vi "Test Bench v14 - TDMS.vi"() -> ()   [LabVIEW 2022 SP3]
uses:
  WhiteNoise.ctl
  <vilib>/Utility/error.llb/DialogType.ctl
  <vilib>/Platform/TimedLoop/XDataNode/timing_clust.ctl
  <vilib>/Platform/TimedLoop/XDataNode/nitl_modes.ctl
  <vilib>/Platform/TimedLoop/XDataNode/wakeup.ctl
  <vilib>/DAQmx/write.llb/DAQmx Write (Analog 2D DBL NChan NSamp).vi
  <vilib>/DAQmx/read.llb/DAQmx Read (Analog 1D DBL 1Chan NSamp).vi
  <vilib>/DAQmx/create/channels.llb/DAQmx Create Channel (AI-Acceleration-Accelerometer).vi
  <vilib>/DAQmx/create/channels.llb/DAQmx Create Channel (AO-Voltage-Basic).vi
  <vilib>/DAQmx/configure/timing.llb/DAQmx Timing (Sample Clock).vi
  <vilib>/DAQmx/miscellaneous.llb/DAQmx Fill In Error Info.vi
  <vilib>/Platform/TimedLoop/TimeConversion.llb/rt-milliseconds-to-timestamp.vi
  <vilib>/platform/TimedLoop/XDataNode/XDataNode.xnode
  <resource>/objmgr/daqmx.rc
  <vilib>/measure/NI_MABase.lvlib
  <vilib>/Platform/TimedLoop/XDataNode/XDNodeRunTimeDep.lvlib
panel:
  in  "stop":bool
  out "x/y":dbl
  out "SampClk.Rate":dbl
  out "Accel. 1 Raw":dbl[](graph)
  in  "Enable Display":bool=TRUE
  in  "Folder to save file to":path=path "C:/Users/LAV-UFSC-2023/Documents/LAV-TCC/Dados-Experimentos/Dados-Bancada-LABVIEW"
  out "Output Signal":dynamicdata(graph)
  in  "Accel. 2":bool
  in  "Input":bool=TRUE
  out "New file path":path
  in  "Signal Output\nControl":enum32{"White Noise", "Harmonic"}(tab)
  in  "White Noise\nParameters":T2={"Seed"=0.0, "Standard Deviation"=0.2, "Reset"=FALSE, "Iterator"=1.0, "Seed"=-1, "Lower Cut-Off"=5.0, "Upper Cut-Off"=350.0} {"Upper Cut-Off" min=5.0 max=350.0 step=10.0; "Lower Cut-Off" min=5.0 max=350.0 step=10.0; "Standard Deviation" min=0.001 max=3.0 step=0.05 format="%0.2p"}
  out "dt White Noise":dbl
  in  "Hamonic\nParameters":T3={"Waveform Type"=0, "Frequency"=10.0, "Amplitude"=0.25} {"Frequency" min=5.0 max=350.0 step=10.0 format="%0.2p"; "Waveform Type" items=["Sine Wave", "Triangle Wave", "Square Wave", "Sawtooth Wave"]; "Amplitude" min=0.001 max=0.3 step=0.05 format="%0.2p"}
  out "dt Harmonic":dbl
  in  "Output":bool=TRUE
  # "Filter"
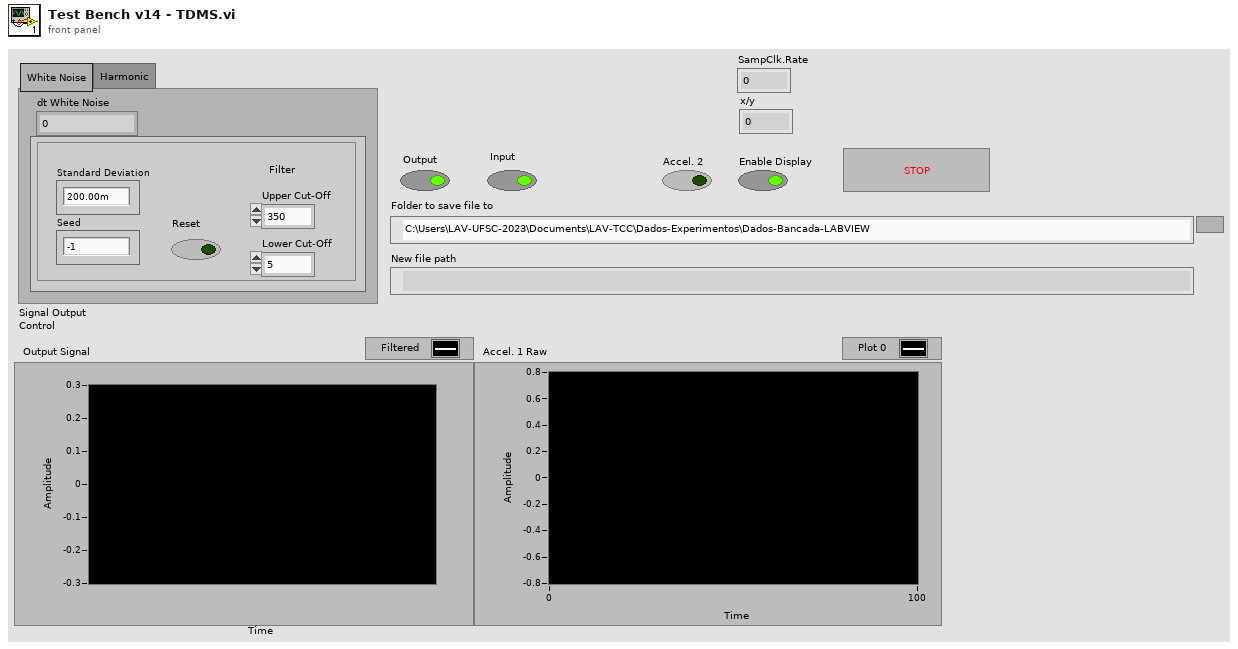
[diagram p1: front panel]
types:
  T1 = typedef "WhiteNoise.ctl" = dbl
  T2 = cluster{"Seed":T1, "Standard Deviation":dbl, "Reset":bool, "Iterator":dbl, "Seed":i8, "Lower Cut-Off":dbl, "Upper Cut-Off":dbl}
  T3 = cluster{"Waveform Type":u16, "Frequency":dbl, "Amplitude":dbl}
  T4 = enum16{"open", "open or create", "create or replace", "create", "open (read-only)"}
  T5 = typedef "DialogType.ctl" = u16
  T6 = typedef "XDNodeRunTimeDep.lvlib/timing_clust.ctl" = cluster{"Expected End [f-1]":u64, "Actual End [f-1]":u64, "Finished Late? [f-1]":bool, "Expected End [i-1]":u64, "Actual End [i-1]":u64, "Finished Late? [i-1]":bool, "Expected Start [i]":u64, "Actual Start [i]":u64, "Expected Start [f]":u64, "Actual Start [f]":u64, "Source Name":string, "Structure Name":string, "Period":i64, "Deadline":i64, "Offset":i64, "Start":i64, "Priority":i32, "Timeout":i32, "Mode":T7, "Wakeup Reason":T8, "Error":errorcluster, "Source Type":string, "Secondary Source Type":string, "Global End Time":u64, "Global Start Time":u64, "Frame Duration":u64, "Iteration Duration":u64, "Assigned CPU":i32, "I/O Scan Engine Mode":u32}
  T7 = typedef "XDNodeRunTimeDep.lvlib/nitl_modes.ctl" = enum32{"No Change", "Process missed periods, maintain original phase", "Discard missed periods, maintain original phase", "Process missed periods, ignore original phase", "Discard missed periods, ignore original phase"}
  T8 = typedef "XDNodeRunTimeDep.lvlib/wakeup.ctl" = enum32{"Normal", "Aborted", "Asynchronous wakeup", "Timing source error", "Timed loop error", "Timeout"}
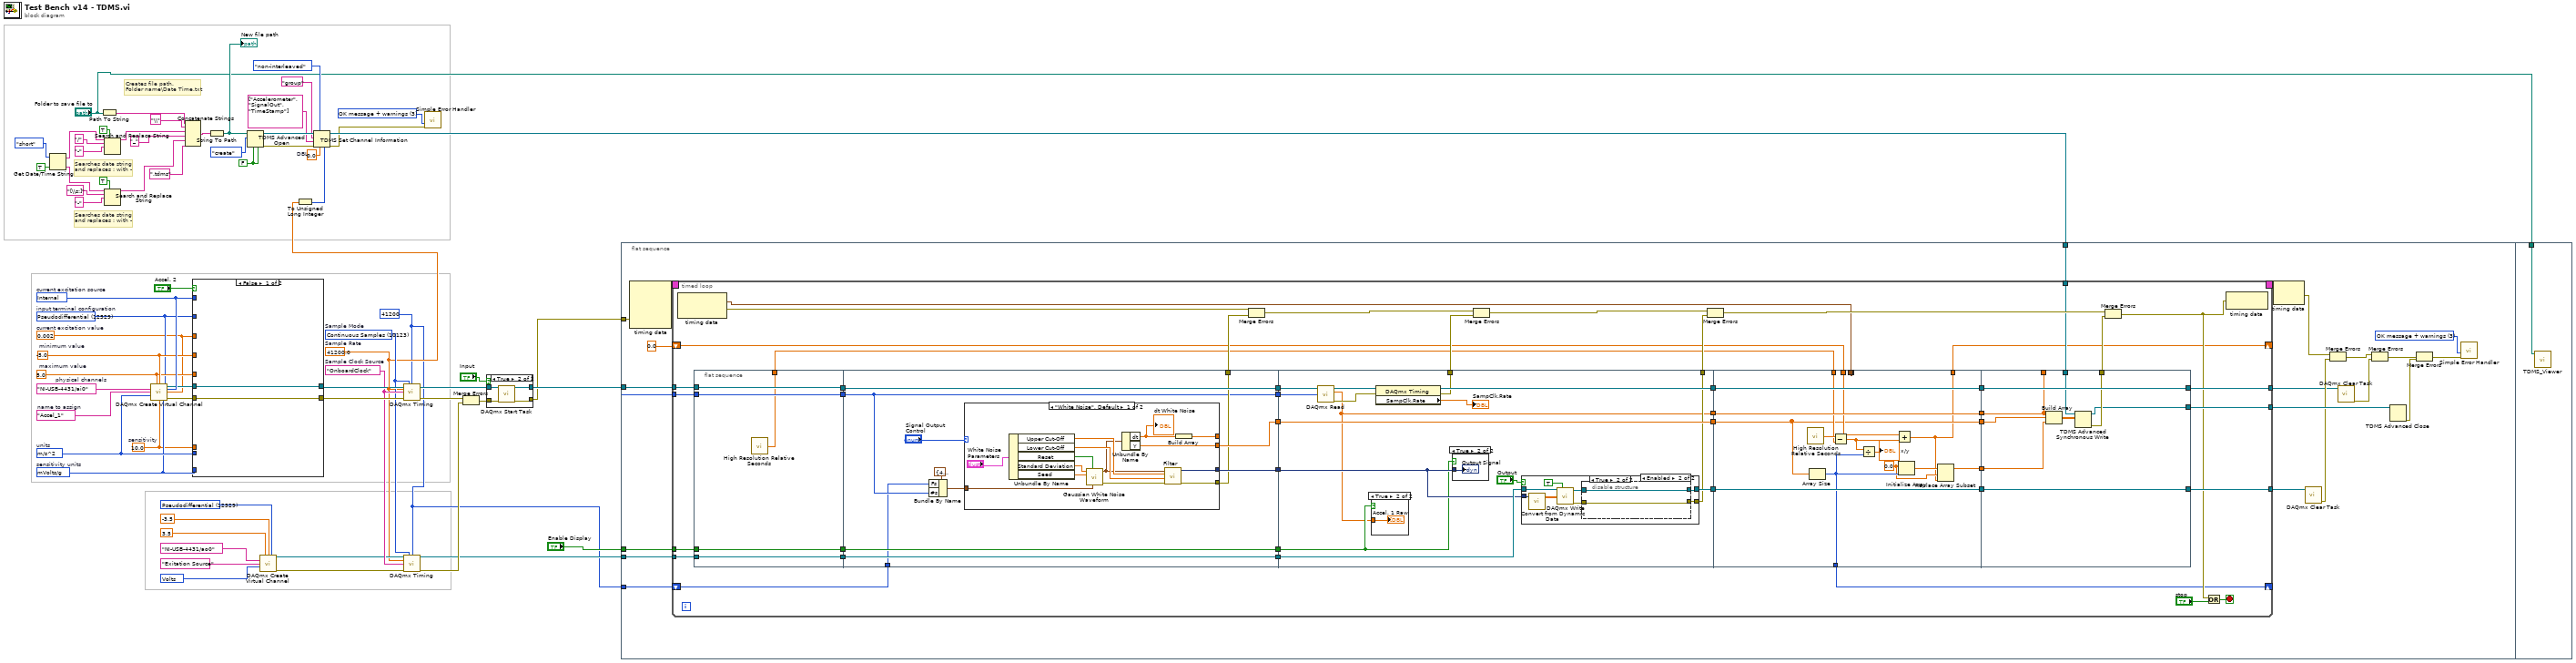
[diagram p0: block diagram]
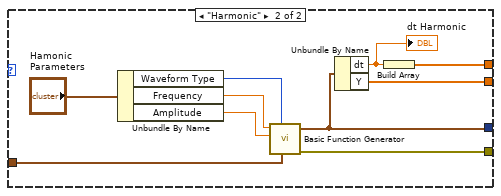
[diagram p2: hidden frame]
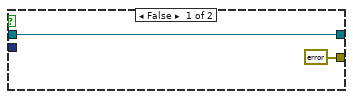
[diagram p5: hidden frame]
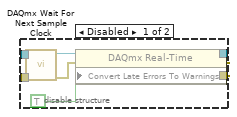
[diagram p6: hidden frame]
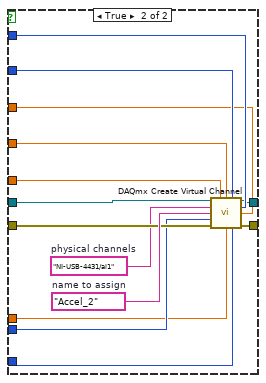
[diagram p7: hidden frame]
diagram:
  w3 = 41200 ("samples per channel")
  w8 = 0.0  # DBL
  w10 = FALSE ("enable asynchronous? (T)")
  w6 = T5 3 items=["no dialog", "OK message", "continue or stop message", "OK message + warnings", "continue/stop + warnings"] ("type of dialog (OK msg:1)")
  w54 = 12529 items=["Default"=-1, "RSE"=10083, "Differential"=10106, "Pseudodifferential"=12529] ("output terminal configuration")
  w52 = 10348 items=["Volts"=10348, "From Custom Scale"=10065] ("units")
  w58 = 12509 items=["mVolts/g"=12509, "Volts/g"=12510]  # sensitivity units
  w48 = 10.0  # sensitivity
  w57 = 0.002  # current excitation value
  w65 = 10200 items=["Internal"=10200, "External"=10167, "None"=10230]  # current excitation source
  w59 = tag "NI-USB-4431/ai0"  # physical channels
  w45 = tag "OnboardClock"  # Sample Clock Source
  w4 = 41200.0  # Sample Rate
  w44 = 10123 items=["Finite Samples"=10178, "Continuous Samples"=10123, "Hardware Timed Single Point"=12522]  # Sample Mode
  w61 = 12529 items=["default"=-1, "RSE"=10083, "NRSE"=10078, "Differential"=10106, "Pseudodifferential"=12529]  # input terminal configuration
  w64 = -5.0  # minimum value
  w63 = 5.0  # maximum value
  w67 = "Accel_1"  # name to assign
  w62 = 12470 items=["g"=10186, "m/s^2"=12470, "in/s^2"=12471, "From Custom Scale"=10065]  # units
  # "Searches date string\nand replaces : with -"
  # "Searches date string\nand replaces : with -"
  # "Creates file path.\nFolder name\\Date Time.txt"
  n1 = Get Date/Time String(date format (0)=enum16{"short", "long", "abbreviated"}."short", want seconds? (F)=TRUE) -> (date string=w18:string, time string=w31:string)  [unwired: 1 in]
  n2 = Path To String(path="Folder to save file to") -> (string=w26:string)
  n3 = Search and Replace String(replace all?=TRUE ("replace all? (F)"), input string=w18, search string="/" ("replace string (\"\")"), replace string="-" ("replace string (\"\")")) -> (result string=w17:string)  [unwired: 4 in, 3 out]
  n4 = Search and Replace String(replace all?=TRUE ("replace all? (F)"), input string=w31, search string="[\\s:]" ("replace string (\"\")"), replace string="-" ("replace string (\"\")")) -> (result string=w24:string)  [unwired: 4 in, 3 out]
  n5 = call-poly <vilib>:"DAQmx Create Virtual Channel.vi"("maximum value"=w63, "minimum value"=w64, "input terminal configuration"=w61, "physical channels"=w59, "current excitation source"=w65, "name to assign"=w67, "current excitation value"=w57, "units"=w62, "sensitivity"=w48, "sensitivity units"=w58) -> ("task out"=w60:refnum<k21>, "error out"=w66:errorcluster)  [unwired: 4 in]
  n6 = Concatenate Strings(w26, "\\" ("string"), w17, "_" ("string"), w24, ".tdms" ("string")) -> (w22:string)
  n7 = case shown="False" "Accel. 2" {
    tunnel: w66 -> [w69 w82]
    tunnel: w65 -> [_ w81]
    tunnel: w64 -> [_ w80]
    tunnel: w63 -> [_ w79]
    tunnel: w62 -> [_ w78]
    tunnel: w61 -> [_ w77]
    tunnel: w60 -> [w68 w76]
    tunnel: w58 -> [_ w74]
    tunnel: w57 -> [_ w73]
    tunnel: w48 -> [_ w72]
    tunnel: [w69 w71] -> w47
    tunnel: [w68 w70] -> w46
    frame False {
    }
    frame True {
      w75 = tag "NI-USB-4431/ai1"  # physical channels
      w83 = "Accel_2"  # name to assign
      n8 = call-poly <vilib>:"DAQmx Create Virtual Channel.vi"("task in"=w76, "maximum value"=w79, "minimum value"=w80, "input terminal configuration"=w77, "physical channels"=w75, "current excitation source"=w81, "name to assign"=w83, "current excitation value"=w73, "units"=w78, "error in"=w82, "sensitivity"=w72, "sensitivity units"=w74) -> ("task out"=w70:refnum<k21>, "error out"=w71:errorcluster)  [unwired: 2 in]
    }
  }
  n9 = String To Path(string=w22) -> (path=w35:path)
  "New file path" <- w35
  n10 = TDMS Advanced Open(4:w10, 6:w10, 10:T4."create" ("operation (0:open)"), 11:w35) -> (0:w14:errorcluster, 3:w13:refnum<k34>)  [unwired: 1 in, 1 out]
  n11 = call-poly <vilib>:"DAQmx Create Virtual Channel.vi"("maximum value"=3.5, "minimum value"=-3.5, "output terminal configuration"=w54, "physical channels"=tag "NI-USB-4431/ao0", "name to assign"="Exitation Source", "units"=w52) -> ("task out"=w42:refnum<k21>, "error out"=w43:errorcluster)  [unwired: 8 in]
  n12 = To Unsigned Long Integer(number=w4) -> (unsigned 32bit integer=w5:u32)
  n13 = TDMS Set Channel Information(4:w5, 6:w8, 7:enum16{"non-interleaved", "interleaved"}."non-interleaved" ("data layout (0:non-interleaved)"), 8:w14, 9:string[] ["Accelerometer", "SignalOut", "TimeStamp"] ("channel name(s)"), 10:"group" ("group name (Untitled)"), 11:w13) -> (0:w7:errorcluster, 3:w34:refnum<k34>)
  n14 = call-poly <vilib>:"DAQmx Timing.vi"("task/channels in"=w46, "sample mode"=w44, "samples per channel"=w3, "rate"=w4, "source"=w45, "error in"=w47) -> ("task out"=w50:refnum<k21>, "error out"=w51:errorcluster)  [unwired: 8 in]
  n15 = call-poly <vilib>:"DAQmx Timing.vi"("task/channels in"=w42, "sample mode"=w44, "samples per channel"=w3, "rate"=w4, "source"=w45, "error in"=w43) -> ("task out"=w40:refnum<k21>, "error out"=w41:errorcluster)  [unwired: 8 in]
  n16 = call <vilib>:"Simple Error Handler.vi"("type of dialog (OK msg:1)"=w6, "error in (no error)"=w7) -> ()  [unwired: 3 in, 5 out]
  n17 = Merge Errors(w51, w41) -> (w36:errorcluster)
  n18 = case shown="True" "Input" {
    tunnel: [w84 w86] -> w37
    tunnel: [w85 w87] -> w2
    tunnel: w36 -> [w85 w88]
    tunnel: w50 -> [w84 w89]
    frame False {
    }
    frame True {
      n19 = call <vilib>:"DAQmx Start Task.vi"("task/channels in"=w89, "error in"=w88) -> ("task out"=w86:refnum<k21>, "error out"=w87:errorcluster)  [unwired: 12 in]
    }
  }
  n20 = flat-sequence {
    tunnel: w40 -> [w106]
    tunnel: w37 -> [w104]
    tunnel: w34 -> [w103]
    tunnel: "Enable Display" -> [w101]
    tunnel: w3 -> [w99]
    tunnel: w2 -> [w92]
    tunnel: "Folder to save file to" -> [w266]
    frame #0 {
      w107 = T5 3 items=["no dialog", "OK message", "continue or stop message", "OK message + warnings", "continue/stop + warnings"] ("type of dialog (OK msg:1)")
      n21 = node-c288(w92) -> (w109:T6)  [unwired: 3 in]
      n22 = timed-loop {
        tunnel: w106 -> [w153]
        tunnel: [w151] -> w105
        tunnel: w104 -> [w152]
        tunnel: [w150] -> w97
        tunnel: w103 -> [w120]
        tunnel: [w147] -> w102
        tunnel: w101 -> [w149]
        shift-right: [w113] -> _
        shift-left: w99 -> [w125]
        tunnel: w99 -> [w134]
        timing: w109 -> [_]
        timing-out: [_] -> w108
        shift-right: [w112] -> _
        shift-left: 0.0 -> [w115]
        stop <- w126 stop-if-true
        n23 = node-c288() -> (w116:timestamp, w118:errorcluster)  [unwired: 1 in]
        n24 = flat-sequence {
          tunnel: w149 -> [w163]
          tunnel: w152 -> [w164]
          tunnel: w153 -> [w165]
          tunnel: [w165] -> w148
          tunnel: [w164] -> w146
          tunnel: [w163] -> w137
          tunnel: w134 -> [w162]
          tunnel: [w162] -> w133
          tunnel: [w161] -> w114
          tunnel: w148 -> [w172]
          tunnel: [w173] -> w145
          tunnel: [w169] -> w143
          tunnel: w146 -> [w173]
          tunnel: [w172] -> w141
          tunnel: [w170] -> w139
          tunnel: [w171] -> w138
          tunnel: w137 -> [w170]
          tunnel: [w167] -> w135
          tunnel: w133 -> [w167]
          tunnel: [w168] -> w132
          tunnel: w125 -> [w166]
          tunnel: w145 -> [w207]
          tunnel: [w201] -> w144
          tunnel: w143 -> [w215]
          tunnel: [w215] -> w142
          tunnel: w141 -> [w213]
          tunnel: [w212] -> w140
          tunnel: w139 -> [w208]
          tunnel: w138 -> [w211]
          tunnel: [w206] -> w136
          tunnel: w135 -> [w205]
          tunnel: [w204] -> w130
          tunnel: [w203] -> w129
          tunnel: w144 -> [w249]
          tunnel: w142 -> [w244]
          tunnel: w140 -> [w251]
          tunnel: w136 -> [w250]
          tunnel: [w251] -> w124
          tunnel: [w250] -> w123
          tunnel: [w249] -> w122
          tunnel: [w244] -> w121
          tunnel: [w248] -> _
          tunnel: w116 -> [w248]
          tunnel: w115 -> [w245]
          tunnel: w114 -> [w246]
          tunnel: [w242] -> w113
          tunnel: [w238] -> w112
          tunnel: [w239] -> w111
          tunnel: [w255] -> w147
          tunnel: [w259] -> w150
          tunnel: [w260] -> w151
          tunnel: w124 -> [w260]
          tunnel: w123 -> [w259]
          tunnel: w122 -> [w253]
          tunnel: w121 -> [w254]
          tunnel: w120 -> [w257]
          tunnel: [w256] -> w119
          tunnel: [w253] -> _
          tunnel: w111 -> [w252]
          frame #0 {
            n25 = call <vilib>:"High Resolution Relative Seconds.vi"() -> ("relative seconds"=w161:dbl)
          }
          frame #1 {
            n26 = Bundle By Name(cluster=cluster{"Fs":dbl, "#s":dbl} {"Fs"=41200.0, "#s"=41200.0} ("sampling info"), "Fs"=w166, "#s"=w167) -> (w175:cluster{"Fs":dbl, "#s":dbl})
            n27 = case shown="\"White Noise\", Default" "Signal Output\nControl" {
              tunnel: [w189 w200] -> w168
              tunnel: w175 -> [w187 w198]
              tunnel: [w179 w193] -> _
              tunnel: [w178 w192] -> w171
              tunnel: [w177 w191] -> w169
              frame "White Noise", Default {
                n28 = Unbundle By Name("White Noise\nParameters") -> ("Upper Cut-Off"=w183:dbl, "Lower Cut-Off"=w182:dbl, "Reset"=w184:bool, "Standard Deviation"=w185:dbl, "Seed"=w186:T1)
                n29 = call <vilib>:"Gaussian White Noise Waveform.vi"("sampling info"=w187, "reset signal"=w184, "seed"=w186, "standard deviation"=w185) -> ("error out"=w190:errorcluster, "signal out"=w181:waveform(dbl))  [unwired: 6 in]
                n30 = Unbundle By Name(w181) -> ("dt"=w180:dbl, "Y"=w177:dbl[])
                "dt White Noise" <- w180
                n31 = call "Filter"("error in (no error)"=w190, "Lower Cut-Off"=w182, "Upper Cut-Off"=w183, "Signal"=w181) -> ("error out"=w189:errorcluster, "Filtered Signal"=w178:dynamicdata)  [unwired: 6 in]
                n32 = Build Array(w180) -> (w179:dbl[])
              }
              frame "Harmonic" {
                n33 = Unbundle By Name("Hamonic\nParameters") -> ("Waveform Type"=w197:u16, "Frequency"=w196:dbl, "Amplitude"=w195:dbl)
                n34 = call <vilib>:"Basic Function Generator.vi"("sampling info"=w198, "signal type"=w197, "amplitude"=w195, "frequency"=w196) -> ("error out"=w200:errorcluster, "signal out"=w192:waveform(dbl))  [unwired: 5 in, 1 out]
                n35 = Unbundle By Name(w192) -> ("dt"=w194:dbl, "Y"=w191:dbl[])
                "dt Harmonic" <- w194
                n36 = Build Array(w194) -> (w193:dbl[])
              }
            }
          }
          frame #2 {
            n37 = call-poly <vilib>:"DAQmx Read.vi"("task/channels in"=w207, "number of samples per channel"=w205) -> ("task out"=w209:refnum<k21>, "data"=w201:dbl[], "error out"=w210:errorcluster)  [unwired: 11 in]
            n38 = case shown="True" w208 {
              tunnel: w201 -> [_ w216]
              frame False {
              }
              frame True {
                "Accel. 1 Raw" <- w216
              }
            }
            n39 = property class="DAQmx Timing"(reference=w209, error in=w210) -> (reference out=w206:refnum<k21>, error out=w204:errorcluster, "SampClk.Rate"=→"SampClk.Rate":dbl)
            n40 = case shown="True" w208 {
              tunnel: w211 -> [_ w217]
              frame False {
              }
              frame True {
                "Output Signal" <- w217
              }
            }
            n41 = case shown="True" "Output" {
              tunnel: w213 -> [w219 w227]
              tunnel: [errorcluster {"status"=FALSE, "code"=0, "source"=""} ("error out") w223] -> w203
              tunnel: [w219 w224] -> w212
              tunnel: w211 -> [_ w222]
              frame False {
              }
              frame True {
                n42 = call "Convert from Dynamic Data"("Dynamic Data Type"=w222) -> ("Array"=w221:dbl[][])  [unwired: 3 in]
                n43 = call-poly <vilib>:"DAQmx Write.vi"("task/channels in"=w227, "auto start"=TRUE, "data"=w221) -> ("task out"=w226:refnum<k21>, "error out"=w225:errorcluster)  [unwired: 10 in, 1 out]
                n44 = disable-structure shown="Enabled" {
                  disable-tunnel: w226 -> [w234 w235]
                  disable-tunnel: w225 -> [w233 w236]
                  disable-tunnel: [w231 w235] -> w224
                  disable-tunnel: [w230 w236] -> w223
                  frame Disabled {
                    n45 = call <vilib>:"DAQmx Wait For Next Sample Clock.vi"("task/channels in"=w234, "error in"=w233) -> ("task out"=w232:refnum<k21>, "error out"=w229:errorcluster)  [unwired: 11 in, 1 out]
                    n46 = property class="DAQmx Real-Time"(reference=w232, error in=w229, "Convert Late Errors To Warnings"=TRUE ("ConvLateErrorsToWarnings")) -> (reference out=w231:refnum<k21>, error out=w230:errorcluster)
                  }
                  frame Enabled {
                  }
                }
              }
            }
          }
          frame #3 {
            w240 = 0.0 ("element")
            n47 = call <vilib>:"High Resolution Relative Seconds.vi"() -> ("relative seconds"=w247:dbl)
            n48 = Array Size(array=w244) -> (size(s)=w242:i32)
            n49 = Subtract(x=w247, y=w246) -> (x-y=w243:dbl)
            n50 = Divide(x=w243, y=w242) -> (x/y=→"x/y":dbl)
            n51 = Add(x=w245, y=w243) -> (x+y=w238:dbl)
            n52 = Initialize Array(w240, w242) -> (w241:dbl[])
            n53 = Replace Array Subset(array=w241, new element=w238, index=w240) -> (w239:dbl[])
          }
          frame #4 {
            n54 = Build Array(w253, w254, w252) -> (w258:dbl[][])
            n55 = TDMS Advanced Synchronous Write(10:w258, 11:w257) -> (0:w256:errorcluster, 3:w255:refnum<k34>)  [unwired: 1 in]
          }
        }
        n56 = Merge Errors(w118, w132) -> (w131:errorcluster)
        n57 = Merge Errors(w131, w130) -> (w128:errorcluster)
        n58 = Merge Errors(w128, w129) -> (w127:errorcluster)
        n59 = Merge Errors(w127, w119) -> (w117:errorcluster)
        n60 = Or(x=w117, y="stop") -> (x .or. y?=w126:bool)
        n61 = node-c288(w117) -> ()  [unwired: 1 out]
      }
      n62 = node-c288(w108) -> (w91:errorcluster)
      n63 = call <vilib>:"DAQmx Clear Task.vi"("task in"=w105) -> ("error out"=w100:errorcluster)  [unwired: 14 in]
      n64 = Merge Errors(w91, w100) -> (w96:errorcluster)
      n65 = call <vilib>:"DAQmx Clear Task.vi"("task in"=w97) -> ("error out"=w95:errorcluster)  [unwired: 14 in]
      n66 = Merge Errors(w96, w95) -> (w94:errorcluster)
      n67 = TDMS Advanced Close(11:w102) -> (0:w98:errorcluster)  [unwired: 3 in, 1 out]
      n68 = Merge Errors(w94, w98) -> (w93:errorcluster)
      n69 = call <vilib>:"Simple Error Handler.vi"("type of dialog (OK msg:1)"=w107, "error in (no error)"=w93) -> ()  [unwired: 3 in, 5 out]
    }
    frame #1 {
      n70 = call "TDMS_Viewer.vi"("Data Directory"=w266) -> ()  [unwired: 11 in]
    }
  }
